vi "Write Coded Binary.vi"(8 "error in":errorcluster, 10 "filter":u8, 11 "PAS Data in":refnum<class "PAS Data.lvclass">) -> (0 "error out":errorcluster, 3 "PAS Data out":refnum<class "PAS Data.lvclass">)   [LabVIEW 2014]
uses:
  Main/Controls/pas_data_enum.ctl
  Devices/TE Cooler/Data/TECData.lvclass
  File IO/File Utilities.lvlib
  Cell/PAS Cell Data.lvclass
  PAS Data.lvclass
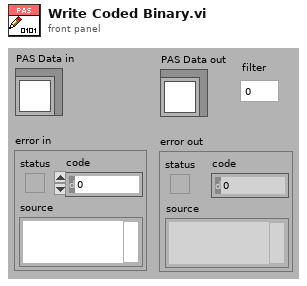
[diagram p1: front panel]
types:
  T1 = typedef "pas_data_enum.ctl" = enum8{"Time", "Ttec", "tecPow", "Spk Position", "Spk Amplification", "Vspan", "Modulation", "Vspk", "Filter", "DC State", "Notes", "O3 Flag", "Raw Flags"}
  T2 = enum16{"big-endian, network order", "native, host order", "little-endian"}
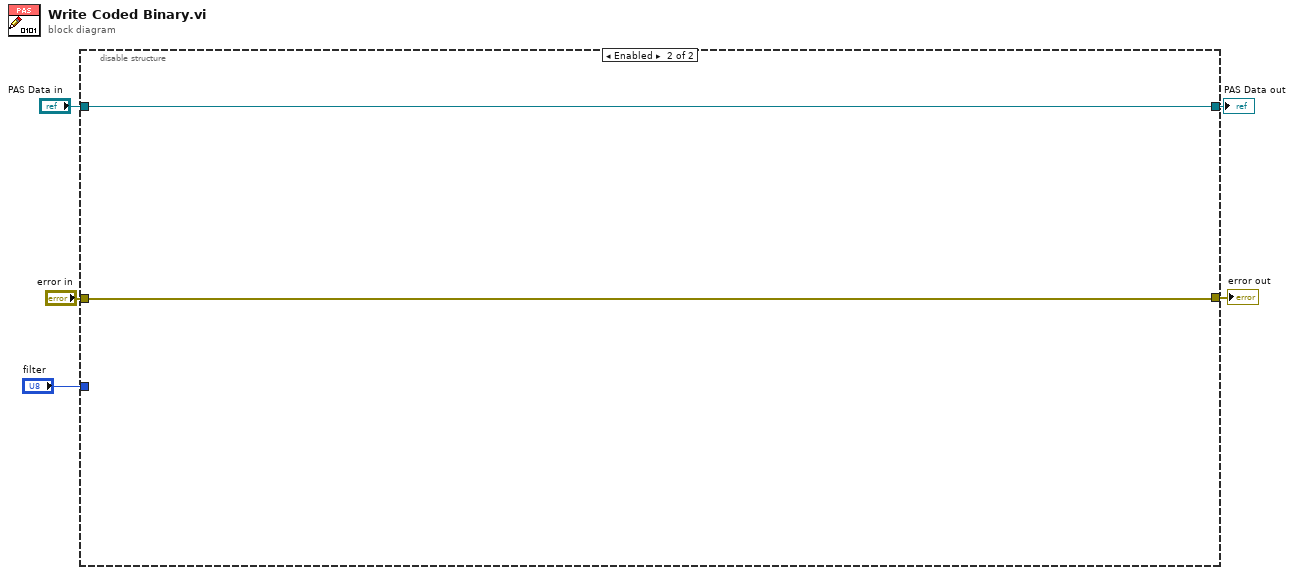
[diagram p0: block diagram]
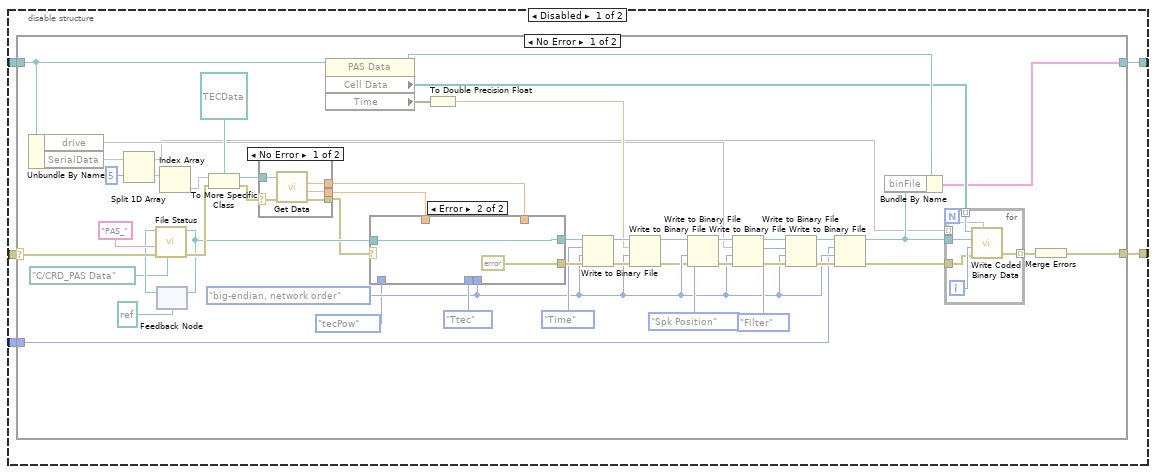
[diagram p2: hidden frame]
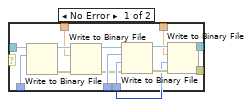
[diagram p3: hidden frame]
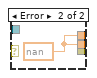
[diagram p4: hidden frame]
diagram:
  n1 = disable-structure shown="Enabled" {
    disable-tunnel: "error in" -> [w10 w89]
    disable-tunnel: [w9 w89] -> w4
    disable-tunnel: "PAS Data in" -> [w8 w90]
    disable-tunnel: [w7 w90] -> w2
    disable-tunnel: "filter" -> [w6 _]
    frame Disabled {
      n2 = case shown="No Error" w10 {
        selector: w10 -> [w35 w88]
        tunnel: [w58 w88] -> w9
        tunnel: [w22 w87] -> w7
        tunnel: w8 -> [w26 w87]
        tunnel: w6 -> [w20 _]
        frame No Error {
          w36 = T2."big-endian, network order" ("byte order (0:big-endian, network order)")
          n3 = Unbundle By Name(w26) -> ("drive"=w44, "SerialData"=w19)
          n4 = Split 1D Array(array=w19, index=5) -> (first subarray=w15:void[], second subarray=w17:void[])
          n5 = feedback #1(refnum<file> refnum ("fileRefOut")) -> (w32:refnum<file>)
          n6 = call "File Status.vi"("Data Path"=path "C:/CRD_PAS Data", "erriorIn"=w35, "prefix"="PAS_", "fileRefIn"=w32) -> ("error out"=w34:errorcluster, "fileRefOut"=w14:refnum<file>)  [unwired: 6 in]
          n7 = feedback-in #1(w14) -> ()
          n8 = Index Array(array=w17) -> (element=w16)  [unwired: 1 in]
          n9 = To More Specific Class(target class=refnum<class "TECData.lvclass"> refnum ("TE Cooler.lvlib:TECData.lvclass"), reference=w16, error in=w34) -> (specific class reference=w46:refnum<class "TECData.lvclass">, error out=w42:errorcluster)
          n10 = case shown="No Error" w42 {
            selector: w42 -> [w76 _]
            tunnel: w46 -> [w79 _]
            tunnel: [w78 w80] -> w45
            tunnel: [w77 _] -> w11
            tunnel: [w75 w80] -> w13
            frame No Error {
              n11 = call "Get Data.vi"("error in (no error)"=w76, "TECData in"=w79) -> ("error out"=w77:errorcluster, "Power"=w75:sgl, "T"=w78:sgl)  [unwired: 6 in, 1 out]
            }
            frame Error {
              w80 = sgl nan ("T")
            }
          }
          n12 = property class="PAS Data"(reference=w26) -> (reference out=w25:refnum<class "PAS Data.lvclass">, "Cell Data"=w23:refnum<class "PAS Cell Data.lvclass">[], "Time"=w24:timestamp)  [unwired: 1 in, 1 out]
          n13 = case shown="Error" w11 {
            tunnel: pas_data_enum."Ttec" ("Enum") -> [w72 _]
            tunnel: [w69 w74] -> w56
            tunnel: [w68 errorcluster {"status"=FALSE, "code"=0, "source"=""} ("error out")] -> w55
            tunnel: w45 -> [w67 _]
            tunnel: w36 -> [w66 _]
            tunnel: w14 -> [w65 w74]
            tunnel: w13 -> [w61 _]
            tunnel: pas_data_enum."tecPow" ("Enum") -> [w59 _]
            frame No Error {
              n14 = Write to Binary File(file (use dialog)=w65, data=w59) -> (refnum out=w64:refnum<file>, error out=w60:errorcluster)  [unwired: 4 in, 1 out]
              n15 = Write to Binary File(file (use dialog)=w64, data=w61, error in=w60) -> (refnum out=w63:refnum<file>, error out=w62:errorcluster)  [unwired: 3 in, 1 out]
              n16 = Write to Binary File(file (use dialog)=w63, data=w72, error in=w62, 9:w66) -> (refnum out=w70:refnum<file>, error out=w71:errorcluster)  [unwired: 2 in, 1 out]
              n17 = Write to Binary File(file (use dialog)=w70, data=w67, error in=w71, 9:w66) -> (refnum out=w69:refnum<file>, error out=w68:errorcluster)  [unwired: 2 in, 1 out]
            }
            frame Error {
            }
          }
          n18 = To Double Precision Float(number=w24) -> (double precision float=w48:dbl)
          n19 = Write to Binary File(file (use dialog)=w56, data=pas_data_enum."Time" ("Enum"), error in=w55, 9:w36) -> (refnum out=w52:refnum<file>, error out=w53:errorcluster)  [unwired: 2 in, 1 out]
          n20 = Write to Binary File(file (use dialog)=w52, data=w48, error in=w53, 9:w36) -> (refnum out=w28:refnum<file>, error out=w27:errorcluster)  [unwired: 2 in, 1 out]
          n21 = Write to Binary File(file (use dialog)=w28, data=pas_data_enum."Spk Position" ("Enum"), error in=w27, 9:w36) -> (refnum out=w50:refnum<file>, error out=w51:errorcluster)  [unwired: 2 in, 1 out]
          n22 = Write to Binary File(file (use dialog)=w50, data=w44, error in=w51, 9:w36) -> (refnum out=w40:refnum<file>, error out=w41:errorcluster)  [unwired: 2 in, 1 out]
          n23 = Write to Binary File(file (use dialog)=w40, data=pas_data_enum."Filter" ("Enum"), error in=w41, 9:w36) -> (refnum out=w39:refnum<file>, error out=w38:errorcluster)  [unwired: 2 in, 1 out]
          n24 = Write to Binary File(file (use dialog)=w39, data=w20, error in=w38, 9:w36) -> (refnum out=w30:refnum<file>, error out=w21:errorcluster)  [unwired: 2 in, 1 out]
          n25 = Bundle By Name(cluster=w25, "binFile"=w30) -> (w22:cluster{})
          n26 = for {
            tunnel: w30 -> [w86]
            tunnel: [w85] -> w43 mode=indexing
            tunnel: w23 -> [w83] mode=indexing
            tunnel: w21 -> [w82]
            tunnel: w15 -> [w81] mode=indexing
            i -> [w84]
            n27 = call-dynamic "Write Coded Binary Data.vi"("AC Data"=w81, "error in"=w82, "cell"=w84, "binRefIn"=w86, "PAS Cell Data in"=w83) -> ("error out"=w85:errorcluster)  [unwired: 5 in, 1 out]
          }
          n28 = Merge Errors(w43) -> (w58:errorcluster)
        }
        frame Error {
        }
      }
    }
    frame Enabled {
    }
  }
  "error out" <- w4
  "PAS Data out" <- w2
